vi "GUI_Bella_Control_Center-ForShowOnly.vi"() -> ()   [LabVIEW 2013]
uses:
  Shared/GUI_Template/GUI_master/tcp new data cluster.ctl
  <vilib>/Analysis/NI_AALBase.lvlib
  <userlib>/_OpenG.lib/numeric/numeric.llb/Random Number Within Range - DBL__ogtk.vi
  Shared/GUI_Template/GUI_master/tcp_new_data_event.ctl
  GUI_TestStand/Fire button.ctl
  Device Drivers/DG645/subVIs/TriggerSource_TypDef.ctl
  Device Driver/LEPS Interface/Filter_typdef.ctl
panel:
  in  "33rd 2":bool
  in  "jklkjljerr 2":bool
  in  "sdfsd 2":bool
  in  "dfggf 2":bool
  in  "33rd":bool
  in  "jklkjljerr":bool
  in  "sdfsd":bool
  in  "dfggf":bool
  in  "GUIdevice 15":string="71146 LEPS Interface"
  in  "filter.var 4::15":T1=enum."Open(6)" caption="Filter Wheel 2"
  in  "filter.var 1::15":T1=enum."Open(6)" caption="Filter Wheel"
  in  "GUIdevice 14":string="PL1-HexCam"
  out "image::14":T2(plugin-control) caption="M1 Cam"
  out "image::13":T2(plugin-control) caption="M1 Cam"
  in  "GUIdevice 13":string="Tel4_Cam"
  out "Trans sigma":dbl=1.7343385167745737 format="%0.2f"
  out "Trans Mean":dbl=100.05882510389497 format="%0.2f"
  out "Waveform Chart":dbl(graph)=100.90190694936402
  out "EnergyIn::12":dbl=20.0 caption="Ein (J)" min=0.0 max=0.0 format="%.1p"
  out "EnergyOut::12":dbl=20.0 caption="Eout (J)" min=0.0 max=0.0 format="%.1p"
  in  "EnergyTransmission::12":dbl=100.0 caption="Etrans (%)" min=0.0 max=0.0
  in  "GUIdevice 12":string="Etrans_Gentecs"
  in  "<command>::1":bool caption="ABORT\nHEXAPOD"
  in  "Step size":dbl=0.01 min=-22.0 max=22.0 format="%.3f"
  in  "Jet trigger":bool caption="Jet Trigger"
  in  "position::9":dbl=41.575 caption="Translation" min=0.0 max=49.0 format="%.3f"
  in  "GUIdevice 9":string="Comp1"
  in  "value::7":dbl=200.0 caption="Bottle (psi)" min=0.0 max=1000.0
  in  "Pressure.device 1::6":dbl=14.35 caption="Line Pressure (psi)" min=15.0 max=314.0 format="%.2f"
  in  "PressureSetPoint.device 2::6":dbl caption="LP line pressure" min=0.0 max=20.0 format="%.2f"
  out "flow::11":dbl caption="Flow (sccm)" min=0.0 max=0.0 format="%.1f"
  in  "valve::11":bool caption="Valve"
  in  "pressure::11":dbl caption="Pressure (Torr)" min=0.0 max=100.0 format="%.2f"
  out "pressure::5":dbl caption="Baratron (Torr)" min=-100.0 max=500.0 format="%.2f"
  in  "Fire Button":T3=TRUE
  in  "Trigger.Source::10":T4=enum."External rising edges" caption="SRS Trigger Mode"
  in  "Delay.Ch C::10":dbl=0.0497 caption="Jet timing (s)" min=-0.1 max=0.1 format="%#_6p"
  in  "position::3":dbl=201.0 caption="position" min=0.0 max=550.0 format="%.1f"
  in  "wangle::1":dbl caption="w (F11 F12)" min=-6.0 max=6.0 step=0.01 format="%_4f"
  in  "vangle::1":dbl caption="v (F9 F10)" min=-6.0 max=6.0 step=0.01 format="%_4f"
  in  "uangle::1":dbl caption="u (F7 F8)" min=-6.0 max=6.0 step=0.01 format="%_4f"
  in  "ypos::1":dbl=3.0 caption="y (F3 F4)" min=-22.0 max=22.0 step=0.01 format="%_4f"
  in  "zpos::1":dbl=-6.0 caption="z (F5 F6)" min=-12.0 max=12.0 step=0.01 format="%_4f"
  in  "xpos::1":dbl=2.0 caption="x (F1 F2)" min=-22.0 max=22.0 step=0.01 format="%_4f"
  in  "stop":bool
  in  "UDP error message":string
  out "Amplitude.Ch CD::10":dbl=0.5 caption="Amplitude Jet trigger" min=0.5 max=5.0
  in  "GUIdevice 7":string="Plasma1_HP_Bottle_Pressure"
  in  "GUIdevice 6":string="PL1-PresCtl"
  in  "GUIdevice 3":string="HPDTelescopeStage"
  in  "parameter::2":string caption="Manual parameter"
  in  "GUIdevice 2":string="BELLA_ManualParameter"
  in  "GUIdevice 1":string="Bella_Hexapod"
  in  "GUIdevice 5":string="BELLA_PDR2000"
  in  "GUIdevice 11":string="BELLA_LowPressureControl"
  out "fire::10":string
  in  "GUIdevice 10":string="BellaSRS"
  out "tcp data event":T5
  out "error IO 2":errorcluster
  # "BELLA CONTROL CENTER"
  # "DELAY GENERATOR"
  # "HEXAPOD"
  # "CAP GAS"
  # "GAS JET"
  # "Target"
  # "ENERGY"
  # "\"-x\" is laser propagation direction"
  # "HPD Stage"
  # "Target"
  # "Compressor"
  # "Target"
  # "Centroid"
  # "Target"
  # "Target"
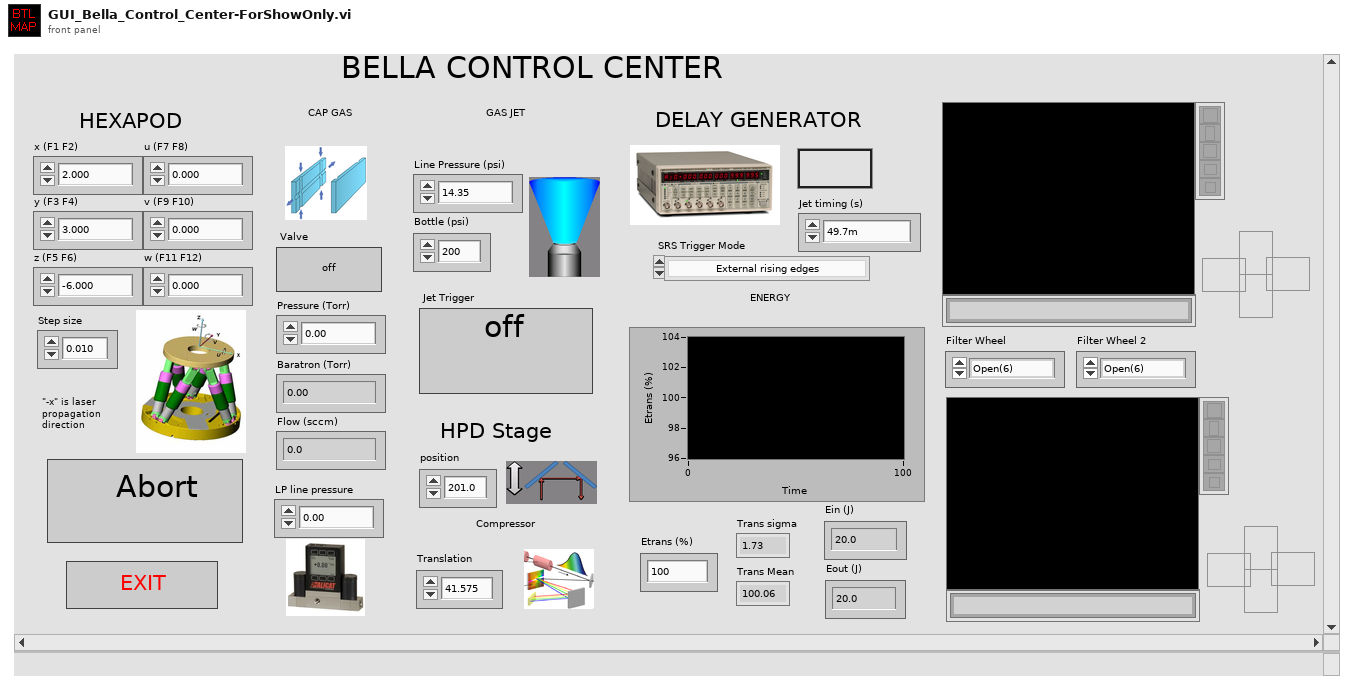
[diagram p1: front panel]
types:
  T1 = typedef "Filter_typdef.ctl" = enum16{"Moving/Unknown", "OD1", "OD2", "OD3", "OD4", "OD5", "Open(6)"}
  T2 = typedef "IMAQ Image.ctl" = refnum<image>
  T3 = typedef "Fire button.ctl" = bool
  T4 = typedef "TriggerSource_TypDef.ctl" = enum16{"Internal", "External rising edges", "External falling edges", "Single shot external rising edges", "Single shot external falling edges", "Single shot", "Line"}
  T5 = typedef "tcp_new_data_event.ctl" = refnum<user-event>
  T6 = typedef "Image Type" = u32
  T7 = typedef "tcp new data cluster.ctl" = cluster{"EventEnum":enum16{"new data", "connection status update"}, "Device name":string}
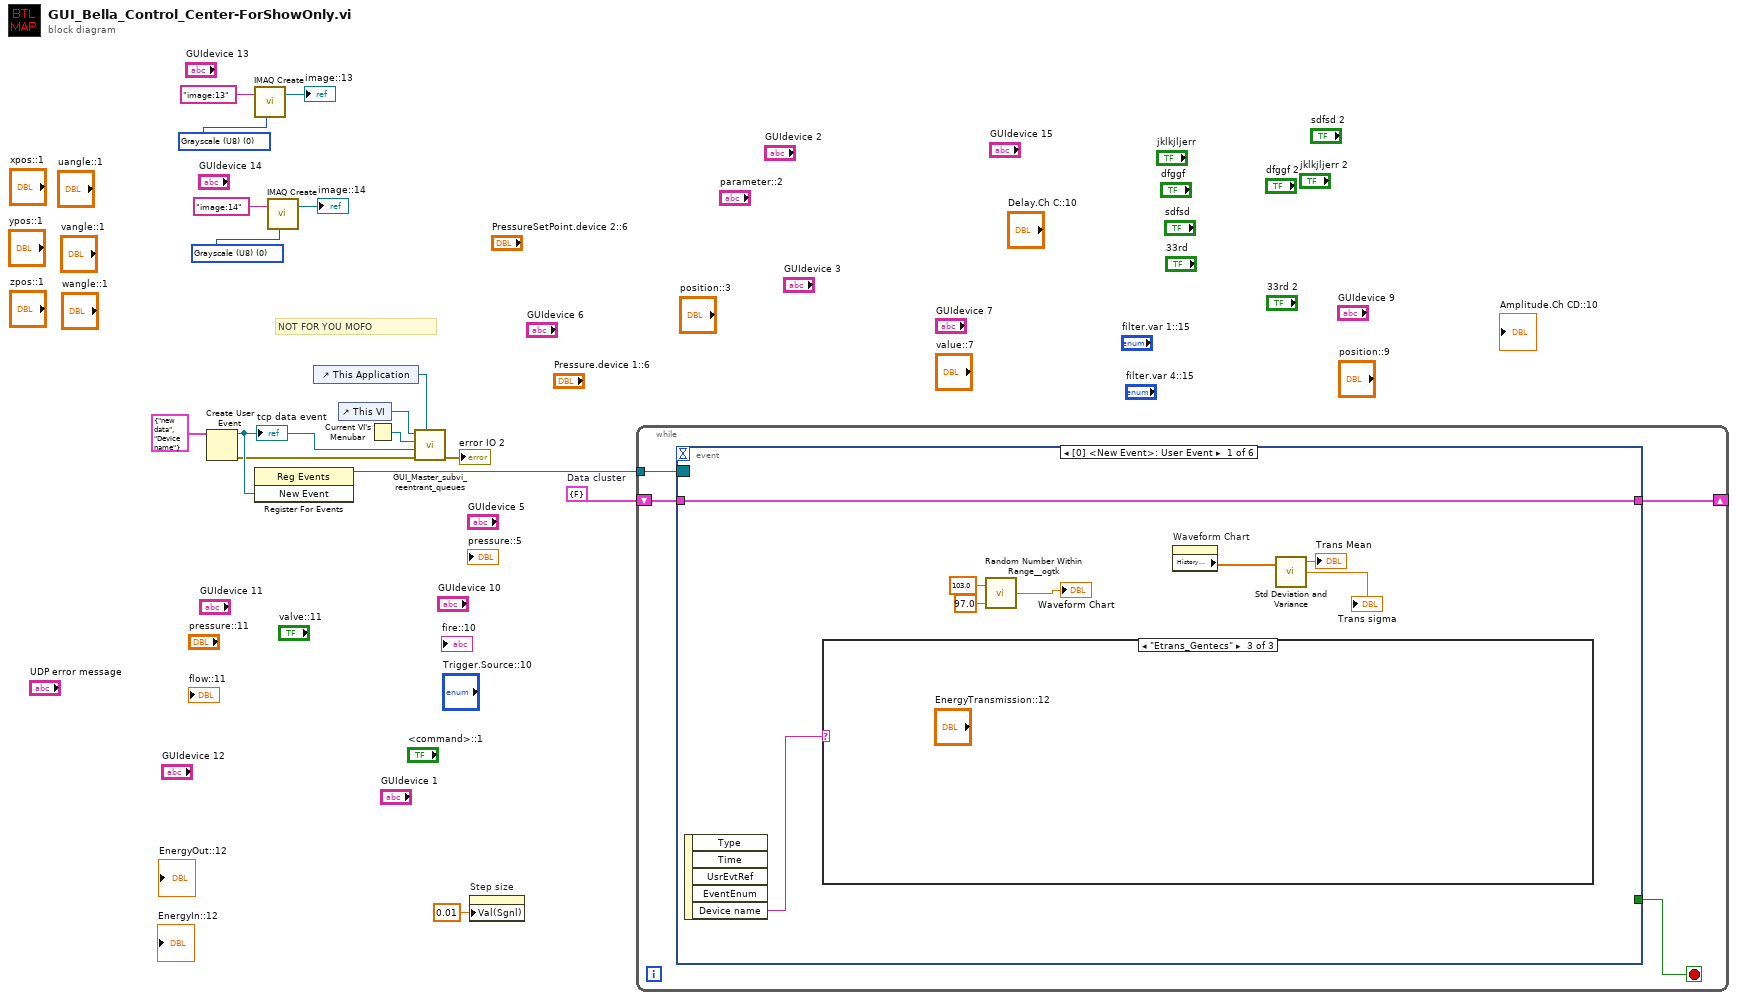
[diagram p0: block diagram]
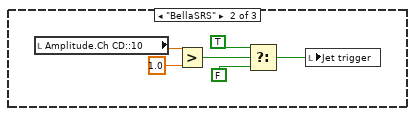
[diagram p3: hidden frame]
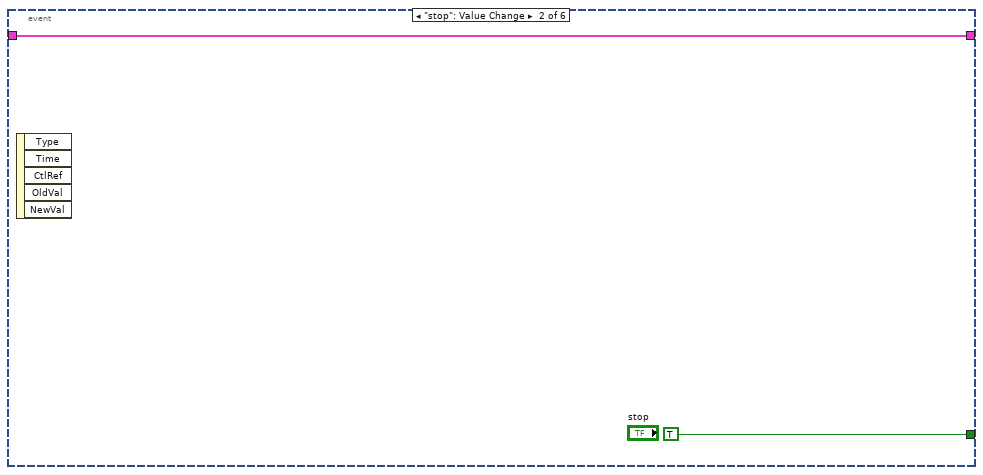
[diagram p4: hidden frame]
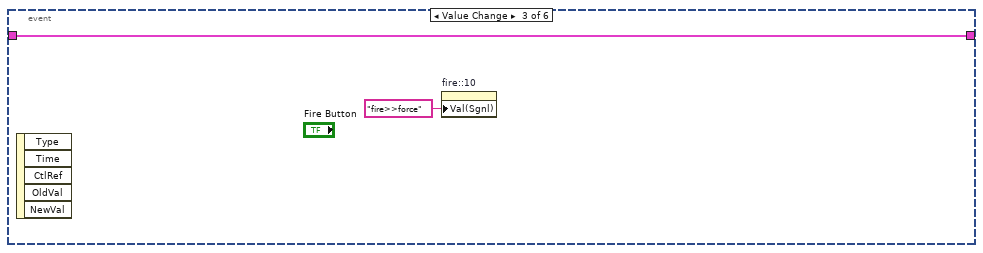
[diagram p5: hidden frame]
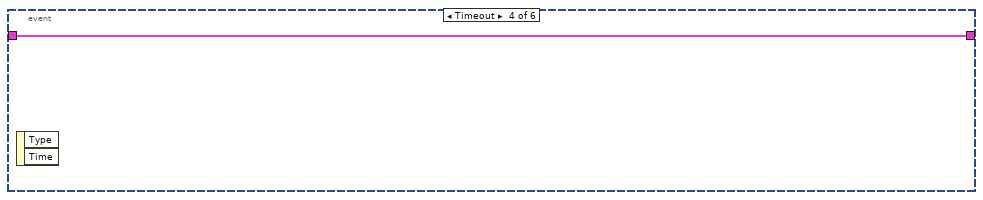
[diagram p6: hidden frame]
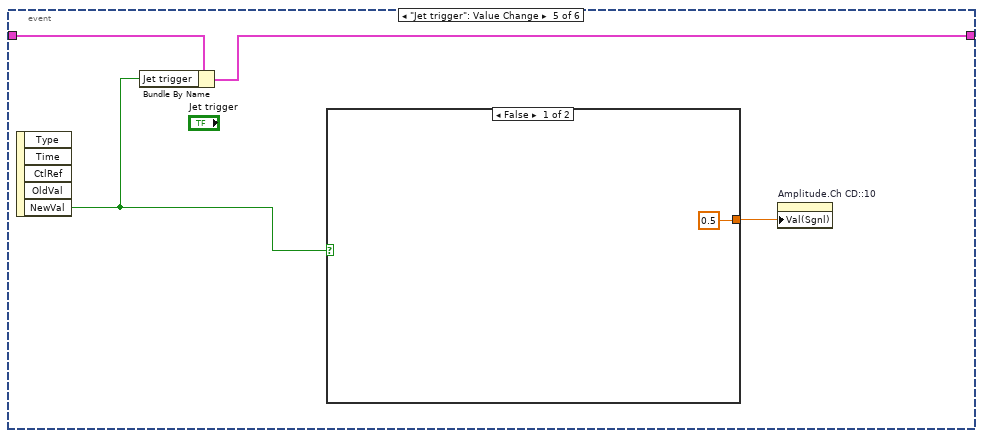
[diagram p7: hidden frame]
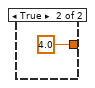
[diagram p8: hidden frame]
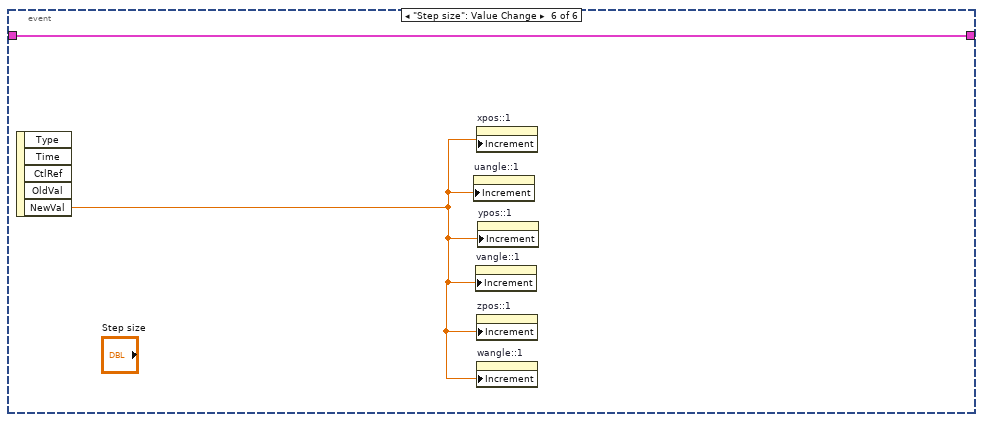
[diagram p9: hidden frame]
diagram:
  w2 = T6 0 items=["Grayscale (U8)", "Grayscale (I16)", "Grayscale (SGL)", "Complex (CSG)", "RGB (U32)", "HSL (U32)", "RGB (U64)", "Grayscale (U16)"] ("Image Type")
  w5 = T6 0 items=["Grayscale (U8)", "Grayscale (I16)", "Grayscale (SGL)", "Complex (CSG)", "RGB (U32)", "HSL (U32)", "RGB (U64)", "Grayscale (U16)"] ("Image Type")
  w7 = cluster{"Jet trigger":bool} {"Jet trigger"=FALSE}  # Data cluster
  # "NOT FOR YOU MOFO"
  n1 = Create User Event(user event datatype=T7 {"EventEnum"=enum."new data", "Device name"="Device name"} ("New Event")) -> (user event=w15:refnum<user-event>, error out=w14:errorcluster)  [unwired: 1 in]
  "tcp data event" <- w15
  n2 = call "IMAQ Create"("Image Name"="image:13", "Image Type"=w5) -> ("New Image"=→"image::13":T2)  [unwired: 3 in, 1 out]
  n3 = register-events(w15) -> (reference out=w10:refnum<event-registration>)  [unwired: 2 in, 1 out]
  n4 = call "IMAQ Create"("Image Name"="image:14", "Image Type"=w2) -> ("New Image"=→"image::14":T2)  [unwired: 3 in, 1 out]
  n5 = control-ref of="This Application"() -> (w16:refnum<vi>)
  n6 = control-ref of="This VI"() -> (w11:refnum<vi>)
  n7 = Current VI's Menubar() -> (w12:refnum<k9>)
  n8 = call "GUI_Master_subvi_reentrant_queues.vi"("This Application"=w16, "error in (no error)"=w14, "tcp data event"=w15, "Caller menu reference"=w12, "Caller VI ref"=w11) -> ("error out"=→"error IO 2":errorcluster)  [unwired: 6 in]
  n9 = property on="Step size" class="DigNum (strict)"("Val(Sgnl)"=0.01 ("Value (Signaling)")) -> ()  [unwired: 2 in, 2 out]
  n10 = while {
    tunnel: w10 -> [w19]
    shift-right: [w17] -> _
    shift-left: w7 -> [w18]
    stop <- w20 stop-if-true
    n11 = event shown="[0] <New Event>: User Event" {
      selector: w19 -> [_ _ _ _ _ _]
      dyn-events: _ -> [_ _ _ _ _ _]
      timeout: _ -> [_ _ _ _ _ _]
      tunnel: [_ TRUE ("stop") _ _ _ _] -> w20
      tunnel: w18 -> [w27 w35 w37 w39 w42 w46]
      tunnel: [w27 w35 w37 w39 w41 w46] -> w17
      event User Event {
        n12 = event-data() -> ("Device name"=w28:string)  [unwired: 1 in, 4 out]
        n13 = case shown="\"Etrans_Gentecs\"" w28 {
          frame "False", Default {
          }
          frame "BellaSRS" {
            n14 = local read "Amplitude.Ch CD::10"() -> (w34:dbl)
            n15 = Greater?(x=w34, y=1.0) -> (0:w32:bool)
            n16 = Select(t=TRUE ("Jet trigger"), s=w32, f=FALSE ("Jet trigger")) -> (s? t:f=w31:bool)
            n17 = local write "Jet trigger"(w31) -> ()
          }
          frame "Etrans_Gentecs" {
          }
        }
        n18 = call-poly <userlib>:"Random Number Within Range__ogtk.vi"("High"=103.0, "Low"=97.0) -> ("Random Number"=→"Waveform Chart":dbl)  [unwired: 3 in]
        n19 = property on="Waveform Chart" class="WFChart (strict)"() -> ("History Data"=w21:dbl[])  [unwired: 2 in, 2 out]
        n20 = call <vilib>:"Std Deviation and Variance.vi"("X"=w21) -> ("mean"=→"Trans Mean":dbl, "standard deviation"=→"Trans sigma":dbl)  [unwired: 1 in, 1 out]
      }
      event "stop": Value Change {
        n21 = event-data() -> ()  [unwired: 1 in, 5 out]
      }
      event Value Change {
        n22 = event-data() -> ()  [unwired: 1 in, 5 out]
        n23 = property on="fire::10" class="Str"("Val(Sgnl)"="fire>>force" ("Value (Signaling)")) -> ()  [unwired: 2 in, 2 out]
      }
      event Timeout {
        n24 = event-data() -> ()  [unwired: 1 in, 2 out]
      }
      event "Jet trigger": Value Change {
        n25 = event-data() -> ("NewVal"=w43:bool)  [unwired: 1 in, 4 out]
        n26 = Bundle By Name(cluster=w42, "Jet trigger"=w43) -> (w41:cluster{"Jet trigger":bool})
        n27 = case shown="False" w43 {
          tunnel: [0.5 ("Amplitude.Ch CD::10") 4.0 ("Amplitude.Ch CD::10")] -> w40
          frame False {
          }
          frame True {
          }
        }
        n28 = property on="Amplitude.Ch CD::10" class="DigNum (strict)"("Val(Sgnl)"=w40) -> ()  [unwired: 2 in, 2 out]
      }
      event "Step size": Value Change {
        n29 = event-data() -> ("NewVal"=w47:dbl)  [unwired: 1 in, 4 out]
        n30 = property on="uangle::1" class="DigNum (strict)"("Increment"=w47) -> ()  [unwired: 2 in, 2 out]
        n31 = property on="vangle::1" class="DigNum (strict)"("Increment"=w47) -> ()  [unwired: 2 in, 2 out]
        n32 = property on="xpos::1" class="DigNum (strict)"("Increment"=w47) -> ()  [unwired: 2 in, 2 out]
        n33 = property on="zpos::1" class="DigNum (strict)"("Increment"=w47) -> ()  [unwired: 2 in, 2 out]
        n34 = property on="wangle::1" class="DigNum (strict)"("Increment"=w47) -> ()  [unwired: 2 in, 2 out]
        n35 = property on="ypos::1" class="DigNum (strict)"("Increment"=w47) -> ()  [unwired: 2 in, 2 out]
      }
    }
  }
